vi "Run Motion Profile.vi"(11 "BufferedTrajectoryPointStream_DevRef":T1) -> ()   [LabVIEW 2019]
uses:
  <vilib>/Rock Robotics/WPI/ThirdParty/Phoenix-LabVIEW/Motor Controller/Controls/CTRE_Phoenix_MotorControl_BufferedTrajectoryPointStream_DeviceRef.ctl
  <vilib>/Rock Robotics/WPI/ThirdParty/Phoenix-LabVIEW/Motor Controller/Controls/CTRE_Phoenix_MotorControl_MotionProfileControlMode.ctl
  RoboRIO/PID.vi
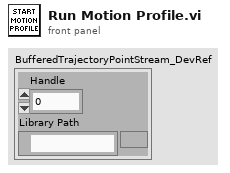
[diagram p1: front panel]
types:
  T1 = typedef "CTRE_Phoenix_MotorControl_BufferedTrajectoryPointStream_DeviceRef.ctl" = cluster{"Handle":u64, "Library Path":path}
  T2 = typedef "CTRE_Phoenix_MotorControl_MotionProfileControlMode.ctl" = u16
  T3 = cluster{"P":dbl, "I":dbl, "D":dbl, "F":dbl, "I Zone":dbl}
  T4 = typedef "WPI_MotorControlDeviceRef.ctl" = cluster{"DeviceStatus":errorcluster, "Type":T5, "PWM":cluster{"PWM Channel":T6, "DeadBand":T7}, "CAN":cluster{"Device Number":u8, "SetOutput VI Ref":variant, "GetOutput VI Ref":variant, "Enable VI Ref":variant, "Disable VI Ref":variant, "Data":variant}, "Invert":bool, "DIO PWM":cluster{"PWM \"Enable\" Channel":T6, "DIOChannel":T8, "PWM Rate":dbl}}
  T5 = typedef "WPI_MotorControlType.ctl" = enum16{"PWM", "CAN", "DIO PWM"}
  T6 = typedef "FPGA_DIOPWMChannel.ctl" = enum8{"PWM 0", "PWM 1", "PWM 2", "PWM 3", "PWM 4", "PWM 5", "PWM 6", "PWM 7", "PWM 8", "PWM 9", "PWM MXP 0", "PWM MXP 1", "PWM MXP 2", "PWM MXP 3", "PWM MXP 4", "PWM MXP 5", "PWM MXP 6", "PWM MXP 7", "PWM MXP 8", "PWM MXP 9", "Invalid"}
  T7 = typedef "WPI_PWMDeadband.ctl" = cluster{"Name":string, "maxPositivePwm":i32, "minPositivePwm":i32, "centerPwm":i32, "maxNegativePwm":i32, "minNegativePwm":i32, "angularRange":u16}
  T8 = typedef "FPGA_DIOChannel.ctl" = enum8{"DIO 0", "DIO 1", "DIO 2", "DIO 3", "DIO 4", "DIO 5", "DIO 6", "DIO 7", "DIO 8", "DIO 9", "DIO MXP 0", "DIO MXP 1", "DIO MXP 2", "DIO MXP 3", "DIO MXP 4", "DIO MXP 5", "DIO MXP 6", "DIO MXP 7", "DIO MXP 8", "DIO MXP 9", "DIO MXP 10", "DIO MXP 11", "DIO MXP 12", "DIO MXP 13", "DIO MXP 14", "DIO MXP 15", "SPI Port CS1", "SPI Port CS2", "SPI Port CS3", "SPI Port MISO", "SPI Port MOSI", "Invalid"}
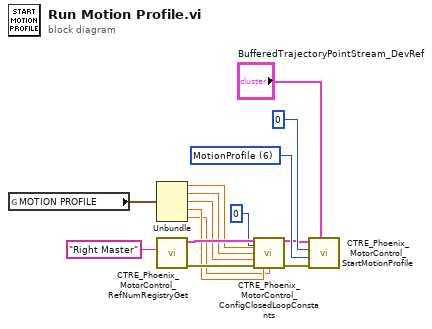
[diagram p0: block diagram]
diagram:
  w14 = T2 6 items=["MotionProfile"=6, "MotionProfileArc"=10] ("Control Mode")
  n1 = global read "PID.vi" "MOTION PROFILE"() -> (w2:T3)
  n2 = Unbundle(w2) -> ("P"=w8:dbl, "I"=w7:dbl, "D"=w6:dbl, "F"=w5:dbl, "I Zone"=w4:dbl)
  n3 = call <vilib>:"CTRE_Phoenix_MotorControl_RefNumRegistryGet.vi"("refnum name"="Right Master") -> ("error out"=w11:errorcluster, "PhoenixMotorControlDevRef"=w12:T4)  [unwired: 9 in]
  n4 = call <vilib>:"CTRE_Phoenix_MotorControl_ConfigClosedLoopConstants.vi"("PhoenixMotorControlDevRef"=w12, "slotIdx"=0, "P"=w8, "I"=w7, "D"=w6, "error in (no error)"=w11, "F"=w5, "I Zone"=w4) -> ("PhoenixMotorControlDevRef"=w10:T4, "error out"=w9:errorcluster)  [unwired: 6 in]
  n5 = call <vilib>:"CTRE_Phoenix_MotorControl_StartMotionProfile.vi"("BufferedTrajectoryPointStream_DevRef"="BufferedTrajectoryPointStream_DevRef", "error in"=w9, "Control Mode"=w14, "minBufferedPts"=u32 0, "PhoenixMotorControlDevRef"=w10) -> ()  [unwired: 5 in, 2 out]
